vi "e.gate HighSpeedPort Decode Buffer.vi"(0 "Data in (binary)":u8[](array[numeric]), 3 "DecodeTimeFormat":string, 7 "error in":errorcluster, 8 "Configuration  in":T1) -> (18 "Configuration out":T1, 23 "data value reference":refnum<data-value>, 24 "data length":i32, 27 "error out":errorcluster)   [LabVIEW 2016]
doc: "This VI is used to decode binary data frames from gantner-instruments e.series controller using configuration cluster information's.\nThe output of the VI is a 2D-array with cells for values and rows for every frame."
uses:
  e.gate Configuration.ctl
  e.gate Channel Data.ctl
  e.gate Data Type.ctl
  e.gate Protocol Type.ctl
  e.gate Module  Data.ctl
  e.gateHSP_DLLhandle.ctl
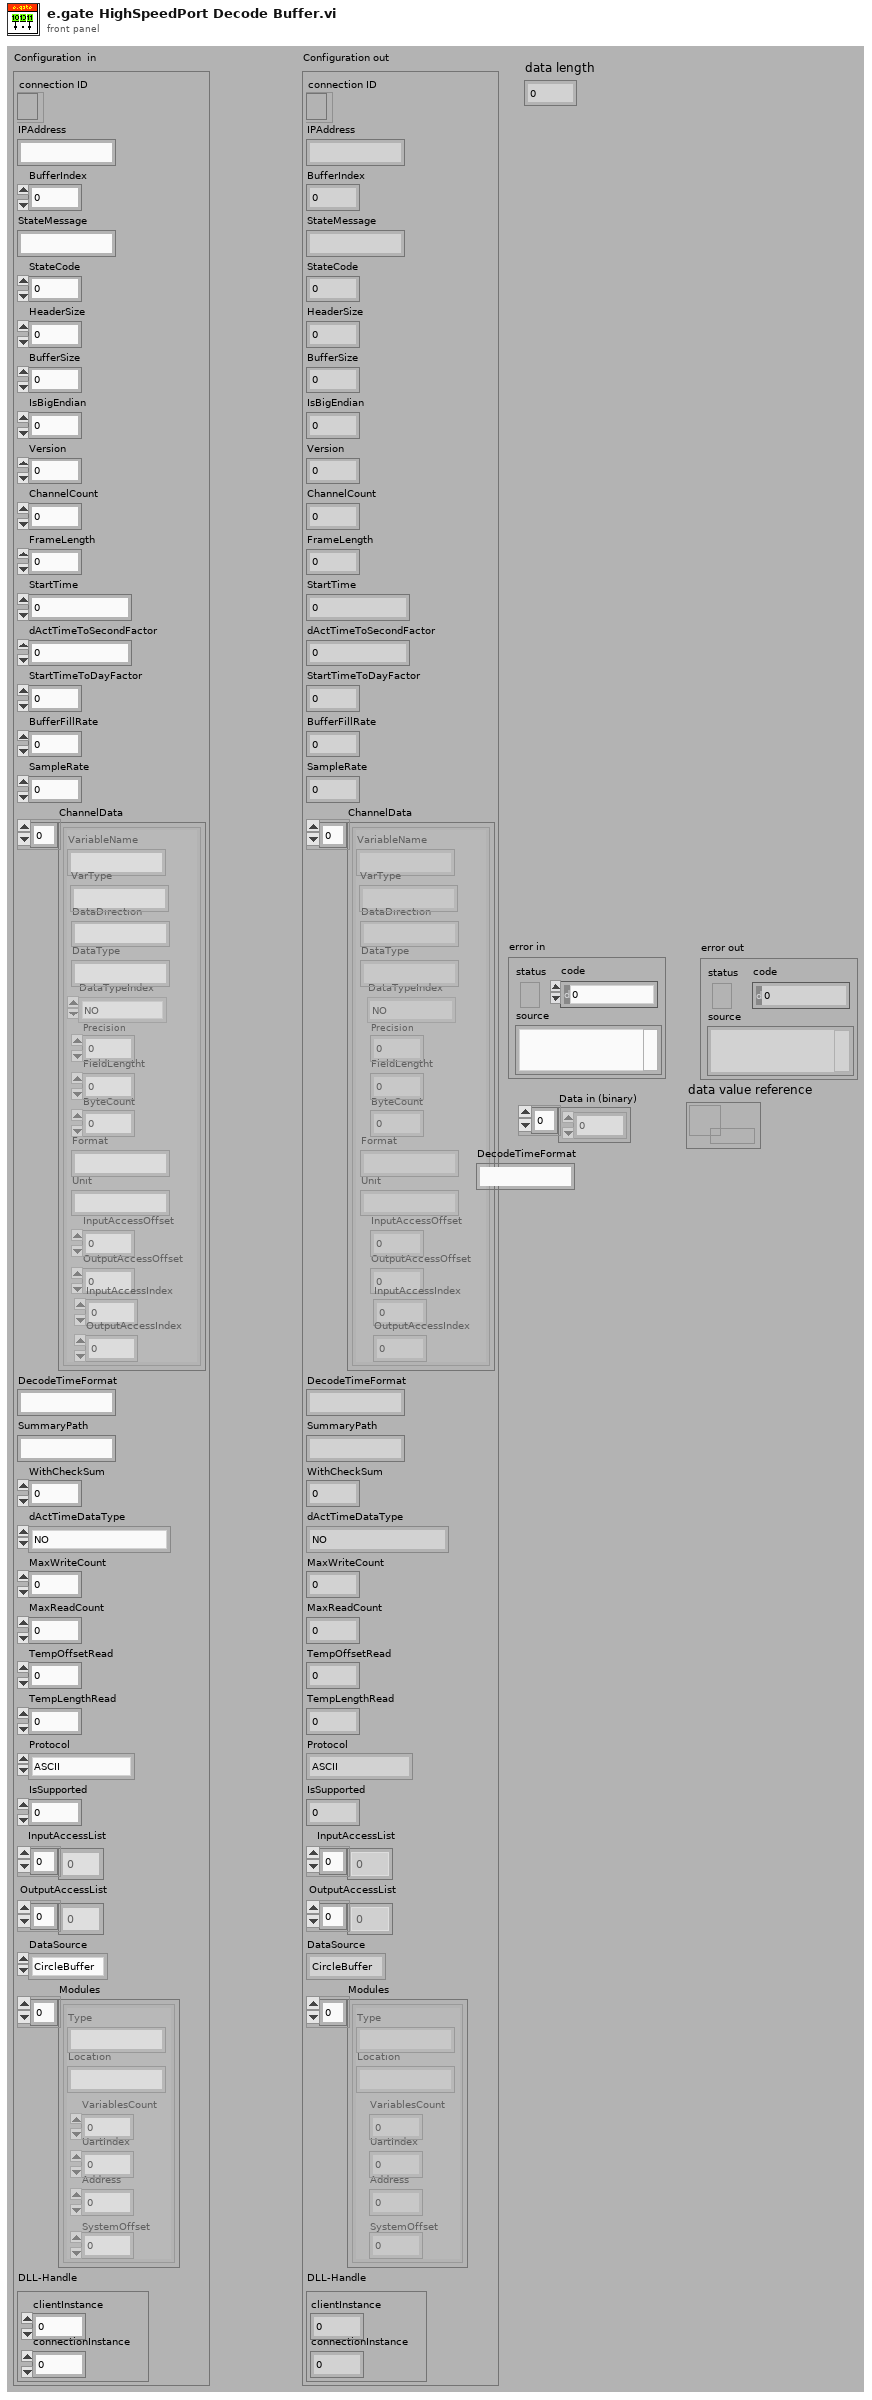
[diagram p1: front panel]
types:
  T1 = typedef "e.gate Configuration.ctl" = cluster{"connection ID":refnum<k5>, "IPAddress":string, "BufferIndex":i32, "StateMessage":string, "StateCode":i8, "HeaderSize":i32, "BufferSize":i32, "IsBigEndian":i32, "Version":i32, "ChannelCount":i32, "FrameLength":i32, "StartTime":dbl, "dActTimeToSecondFactor":dbl, "StartTimeToDayFactor":dbl, "BufferFillRate":dbl, "SampleRate":dbl, "ChannelData":T2[], "DecodeTimeFormat":string, "SummaryPath":string, "WithCheckSum":i32, "dActTimeDataType":T3, "MaxWriteCount":i32, "MaxReadCount":i32, "TempOffsetRead":i32, "TempLengthRead":i32, "Protocol":T4, "IsSupported":i32, "InputAccessList":i32[], "OutputAccessList":i32[], "DataSource":enum16{"CircleBuffer", "test.con Logger", "test.con Archive"}, "Modules":T5[], "DLL-Handle":T6}
  T2 = typedef "e.gate Channel Data.ctl" = cluster{"VariableName":string, "DataDirection":string, "DataType":string, "DataTypeIndex":T3, "Precision":i16, "FieldLengtht":i16, "ByteCount":i32, "Format":string, "Unit":string, "InputAccessOffset":i32, "OutputAccessOffset":i16, "InputAccessIndex":i16, "OutputAccessIndex":i16, "VarType":string}
  T3 = typedef "e.gate Data Type.ctl" = enum16{"NO", "BOOL", "SINT8", "USINT8", "SINT16", "USINT16", "SINT32", "USINT32", "FLOAT", "SET8", "SET16", "SET32", "DOUBLE", "SINT64", "USINT64", "SET64"}
  T4 = typedef "e.gate Protocol Type.ctl" = enum16{"ASCII", "HighspeedPort Online", "HighspeedPort Buffer", "eGateHighspeedPortDLL "}
  T5 = typedef "e.gate Module  Data.ctl" = cluster{"Type":string, "Location":string, "VariablesCount":i16, "UartIndex":i16, "Address":i16, "SystemOffset":i16}
  T6 = typedef "e.gateHSP_DLLhandle.ctl" = cluster{"clientInstance":i32, "connectionInstance":i32}
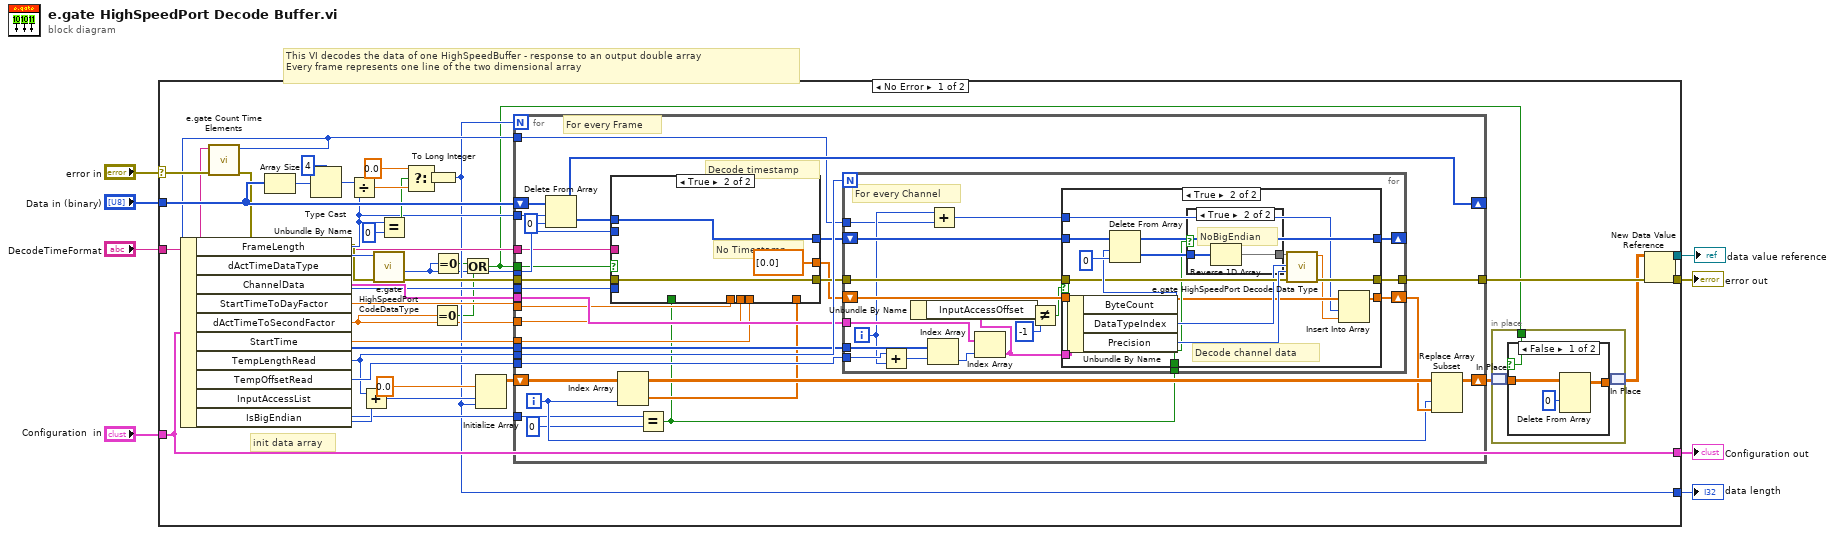
[diagram p0: block diagram]
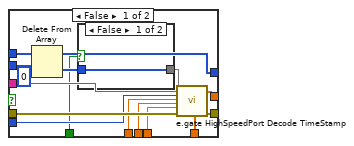
[diagram p3: hidden frame]
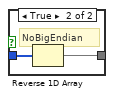
[diagram p4: hidden frame]
diagram:
  # "This VI decodes the data of one HighSpeedBuffer - response to an output double array\nEvery frame represents one line of the two dimensional array"
  n1 = case shown="No Error" "error in" {
    selector: "error in" -> [w25 w148]
    tunnel: "Data in (binary)" -> [w43 _]
    tunnel: "Configuration  in" -> [w40 w147]
    tunnel: [w16 w148] -> w6
    tunnel: [w40 w147] -> w5
    tunnel: "DecodeTimeFormat" -> [w23 _]
    tunnel: [w18 _] -> w2
    tunnel: [w14 _] -> w1
    frame No Error {
      # "init data array"
      n2 = Unbundle By Name(w40) -> ("FrameLength"=w33:i32, "dActTimeDataType"=w30:T3, "ChannelData"=w39:T2[], "StartTimeToDayFactor"=w38:dbl, "dActTimeToSecondFactor"=w13:dbl, "StartTime"=w37:dbl, "TempLengthRead"=w26:i32, "TempOffsetRead"=w31:i32, "InputAccessList"=w29:i32[], "IsBigEndian"=w21:i32)
      n3 = call "e.gate Count Time Elements.vi"("error in (no error)"=w25, "Time Format String"=w23) -> ("error out"=w24:cluster{"status":bool, i32, "source":string}, "NumberOfTimeElements"=w22:i32)  [unwired: 8 in]
      n4 = Array Size(array=w43) -> (size(s)=w45:i32)
      n5 = Type Cast(type=4 ("Länge"), x=w45) -> (*(type *) &x=w46:i32)
      n6 = Divide(x=w46, y=w33) -> (x/y=w36:dbl)
      n7 = Add(x=w26, y=w22) -> (x+y=w20:i32)
      n8 = call "e.gate HighSpeedPort CodeDataType.vi"("error in (no error)"=w24, "TransferDataType"=w30) -> ("error out"=w41:errorcluster, "ByteCount"=w12:i32)  [unwired: 2 in, 6 out]
      n9 = Equal?(x=w33, y=0) -> (x = y?=w34:bool)
      n10 = Select(t=0.0, s=w34, f=w36) -> (s? t:f=w19:dbl)
      n11 = To Long Integer(number=w19) -> (32bit integer=w18:i32)
      n12 = Equal To 0?(x=w13) -> (x = 0?=w10:bool)
      n13 = Equal To 0?(x=w12) -> (x = 0?=w11:bool)
      n14 = Or(x=w11, y=w10) -> (x .or. y?=w9:bool)
      n15 = Initialize Array(0.0 ("Element"), w20, w18) -> (w27:dbl[][])
      n16 = for {
        N: w18 -> [_]
        tunnel: w26 -> [w83]
        shift-right: [w78] -> _
        shift-left: w43 -> [w82]
        tunnel: w33 -> [w77]
        tunnel: [w75] -> w42
        tunnel: w39 -> [w76]
        shift-right: [w63] -> w17
        shift-left: w27 -> [w62]
        tunnel: w12 -> [w69]
        tunnel: w41 -> [w73]
        tunnel: w23 -> [w68]
        tunnel: w30 -> [w72]
        tunnel: w38 -> [w71]
        tunnel: w13 -> [w67]
        tunnel: w37 -> [w70]
        tunnel: w31 -> [w65]
        tunnel: w29 -> [w66]
        tunnel: w22 -> [w58]
        tunnel: w21 -> [w57]
        tunnel: w9 -> [w54]
        i -> [w60]
        # "For every Frame"
        # "Decode timestamp"
        n17 = Delete From Array(array=w82, length=w77, index=0 ("Index")) -> (deleted portion=w80:u8[], array with subset deleted=w78:u8[])
        n18 = Index Array(array=w62, index (col)=w60) -> (element=w59:dbl[])  [unwired: 1 in]
        n19 = Equal?(x=w57, y=0) -> (x = y?=w55:bool)
        n20 = case shown="True" w54 {
          tunnel: w80 -> [w99 w105]
          tunnel: [w98 w105] -> w79
          tunnel: [w97 dbl[] [0.0] ("date time array (double)")] -> w64
          tunnel: [w96 w104] -> w74
          tunnel: w73 -> [w95 w104]
          tunnel: w69 -> [w94 _]
          tunnel: w68 -> [w93 _]
          tunnel: w72 -> [w92 _]
          tunnel: w71 -> [w91 _]
          tunnel: w67 -> [w90 _]
          tunnel: w70 -> [w89 _]
          tunnel: w59 -> [w87 _]
          tunnel: w55 -> [w84 _]
          frame False {
            n21 = Delete From Array(array=w99, length=w94, index=0) -> (deleted portion=w86:u8[], array with subset deleted=w98:u8[])
            n22 = case shown="False" w84 {
              tunnel: w86 -> [w100 w102]
              tunnel: [w100 w101] -> w85
              frame False {
              }
              frame True {
                # "NoBigEndian"
                n23 = Reverse 1D Array(array=w102) -> (reversed array=w101:u8[])
              }
            }
            n24 = call "e.gate HighSpeedPort Decode TimeStamp.vi"("Data in (binary)"=w85, "Time Format String"=w93, "dActTimeDataType"=w92, "StartTimeToDayFactor"=w91, "dActTimeToSecondFactor"=w90, "StartTime"=w89, "error in (no error)"=w95, "Array"=w87) -> ("date time array (double)"=w97:dbl[], "error out"=w96:cluster{"status":bool, i32, "source":string})  [unwired: 18 out]
          }
          frame True {
            # "No Timestamp"
          }
        }
        n25 = for {
          N: w83 -> [_]
          shift-right: [w124] -> _
          shift-left: w79 -> [w123]
          shift-right: [w120] -> w61
          shift-left: w64 -> [w119]
          tunnel: w76 -> [w118]
          tunnel: w74 -> [w121]
          tunnel: [w122] -> w75
          tunnel: w66 -> [w113]
          tunnel: w65 -> [w110]
          tunnel: w58 -> [w107]
          tunnel: w55 -> [w106]
          i -> [w109]
          # "For every Channel"
          n26 = Add(x=w110, y=w109) -> (x+y=w111:i32)
          n27 = Index Array(array=w113, index=w111) -> (element=w112:i32)
          n28 = Add(x=w109, y=w107) -> (x+y=w108:i32)
          n29 = Index Array(array=w118, index=w112) -> (element=w117:T2)
          n30 = Unbundle By Name(w117) -> ("InputAccessOffset"=w115:i32)
          n31 = Not Equal?(x=w115, y=-1) -> (x != y?=w116:bool)
          n32 = case shown="True" w116 {
            tunnel: [w127 w143] -> w124
            tunnel: w123 -> [w127 w142]
            tunnel: [w126 w138] -> w122
            tunnel: w121 -> [w126 w137]
            tunnel: [w125 w128] -> w120
            tunnel: w119 -> [w125 w131]
            tunnel: w117 -> [_ w136]
            tunnel: w108 -> [_ w129]
            tunnel: w106 -> [_ w132]
            frame False {
            }
            frame True {
              # "Decode channel data"
              n33 = Unbundle By Name(w136) -> ("ByteCount"=w140:i32, "DataTypeIndex"=w135:T3, "Precision"=w139:i16)
              n34 = Delete From Array(array=w142, length=w140, index=0 ("Index")) -> (deleted portion=w134:u8[], array with subset deleted=w143:u8[])
              n35 = case shown="True" w132 {
                tunnel: w134 -> [w144 w146]
                tunnel: [w144 w145] -> w133
                frame False {
                }
                frame True {
                  # "NoBigEndian"
                  n36 = Reverse 1D Array(array=w146) -> (reversed array=w145:u8[])
                }
              }
              n37 = call "e.gate HighSpeedPort Decode Data Type.vi"("error in (no errro)"=w137, "Precision"=w139, "DataTypeIndex"=w135, "data in (binary)"=w133) -> ("error out"=w138:errorcluster, "value (double)"=w130:dbl)  [unwired: 6 out]
              n38 = Insert Into Array(array=w131, index=w129, new element=w130) -> (w128:dbl[])
            }
          }
        }
        n39 = Replace Array Subset(array=w62, new element=w61, index (col)=w60) -> (w63:dbl[][])  [unwired: 1 in]
      }
      n40 = in-place {
        in-place-border: w9 -> [w47]
        n41 = in-place-match #1(w17) -> (w49:dbl[][])
        n42 = case shown="False" w47 {
          tunnel: w49 -> [w52 w53]
          tunnel: [w51 w53] -> w48
          frame False {
            n43 = Delete From Array(array=w52, index (row)=0) -> (array with subset deleted=w51:dbl[][])  [unwired: 2 in, 1 out]
          }
          frame True {
            # "No Timestamp"
          }
        }
        n44 = in-place-match #1(w48) -> (w15:dbl[][])
      }
      n45 = New Data Value Reference(data value=w15, error in=w42) -> (data value reference=w14:refnum<data-value>, error out=w16:errorcluster)
    }
    frame Error {
    }
  }
  "data value reference" <- w1
  "error out" <- w6
  "Configuration out" <- w5
  "data length" <- w2
